vi "Do.vi"(8 "error in (no error)":errorcluster, 10 "Actor in":refnum<class "Actor.lvclass">, 11 "Create Test Executive Msg":refnum<class "Create Test Executive Msg.lvclass">) -> (0 "error out":errorcluster, 2 "Actor out":refnum<class "Actor.lvclass">)   [LabVIEW 2017, in "Create Test Executive Msg.lvclass"]
doc: "This VI delivers the message to the actor by calling the appropriate method(s) on the actor."
uses:
  <vilib>/gpm_packages/@cs/Test-executive-builder/Source/Test Executive Builder Model/Test Executive Builder Model Messages/Create Test Executive Msg/Create Test Executive Msg.lvclass
  <vilib>/ActorFramework/Actor/Actor.lvclass
  <vilib>/gpm_packages/@cs/Test-executive-builder/Source/Test Executive Builder Model/Test Executive Builder Model/Test Executive Builder Model.lvclass
  C:/Program Files/National Instruments/LabVIEW 2017/vi.lib/ActorFramework/Actor/Actor.lvclass
  <vilib>/gpm_packages/@cs/Test-executive-builder/Source/Test Executive Builder Model/Test Executive Builder Model Messages/Create Test Executive Msg/Create Test Executive Msg.lvclass/Create Test Executive Msg.ctl
  <vilib>/gpm_packages/@cs/Test-executive-builder/Source/Application Dependencies/Create Test Executive.ctl
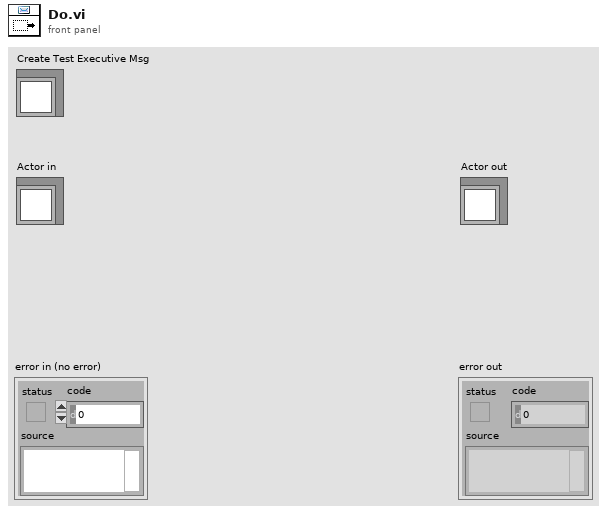
[diagram p1: front panel]
types:
  T1 = typedef "Create Test Executive.ctl" = cluster{"Folder Path":path, "File Name with Extension":string}
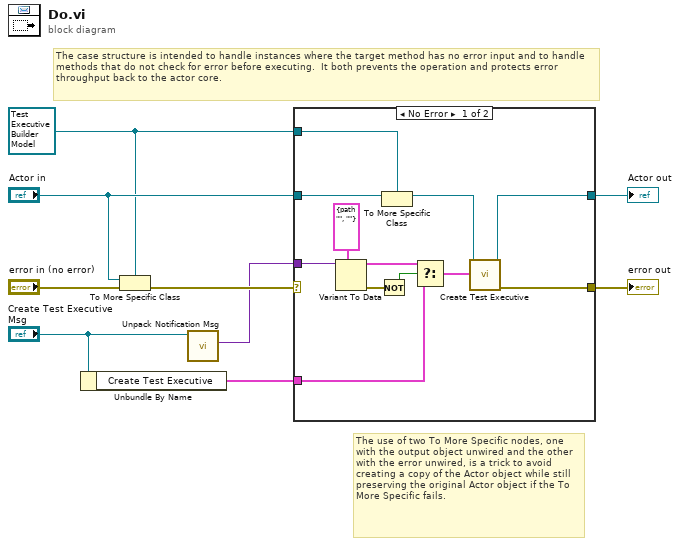
[diagram p0: block diagram]
diagram:
  w4 = refnum<class "Test Executive Builder Model.lvclass"> refnum ("Actor in")
  # "The use of two To More Specific nodes, one with the output object unwired and the other with the error unwired, is a trick to avoid creating a copy of the Actor object while still preserving the original Actor object if the To More Specific fails."
  # "The case structure is intended to handle instances where the target method has no error input and to handle methods that do not check for error before executing.  It both prevents the operation and protects error throughput back to the actor core."
  n1 = Unbundle By Name("Create Test Executive Msg") -> ("Create Test Executive"=w1:T1)
  n2 = To More Specific Class(target class=w4, reference="Actor in", error in="error in (no error)") -> (error out=w8:errorcluster)  [unwired: 1 out]
  n3 = call-dynamic "Unpack Notification Msg.vi"("Notification Msg"="Create Test Executive Msg") -> ("Value"=w3:variant)  [unwired: 8 in, 2 out]
  n4 = case shown="No Error" w8 {
    selector: w8 -> [_ w23]
    tunnel: [w21 w23] -> w7
    tunnel: [w20 w22] -> w6
    tunnel: "Actor in" -> [w19 w22]
    tunnel: w4 -> [w18 _]
    tunnel: w3 -> [w13 _]
    tunnel: w1 -> [w10 _]
    frame No Error {
      n5 = Variant To Data(type=T1 {"Folder Path"=path "", "File Name with Extension"=""} ("Create Test Executive"), Variant=w13) -> (data=w12:T1, error out=w16:errorcluster)  [unwired: 1 in]
      n6 = Not(x=w16) -> (.not. x?=w15:bool)
      n7 = To More Specific Class(target class=w18, reference=w19) -> (specific class reference=w17:refnum<class "Test Executive Builder Model.lvclass">)  [unwired: 1 in, 1 out]
      n8 = Select(t=w12, s=w15, f=w10) -> (s? t:f=w11:T1)
      n9 = call-dynamic "Create Test Executive.vi"("Create Test Executive"=w11, "Test Executive Builder Model in"=w17) -> ("error out"=w21:errorcluster, "Test Executive Builder Model out"=w20:refnum<class "Test Executive Builder Model.lvclass">)  [unwired: 7 in, 1 out]
    }
    frame Error {
      # "If type check fails, pass the original object out again."
    }
  }
  "error out" <- w7
  "Actor out" <- w6
